vi "Configure Trigger.vi"(8 "error in":errorcluster, 11 "object in":refnum<class "Fetch Waveforms CFG.lvclass">) -> (0 "error out":errorcluster, 3 "object out":refnum<class "Fetch Waveforms CFG.lvclass">)   [LabVIEW 2023, in "Scope Simulated CFGs.lvlib" / "Fetch Waveforms CFG.lvclass"]
uses:
  Fetch Waveforms CFG.lvclass
  Configuration/Configuration JSON/Configuration JSON Base/CFG JSON.lvclass/CFG JSON.ctl
  49d2c016-646b-4808-92bd-86f31724cd2e.vi
  <vilib>/JDP Science/JSONtext/Find Item.vi
  <vilib>/JDP Science/JSONtext/Next JSON Value.vi
  <vilib>/JDP Science/JSONtext/String Subset.vi
  <vilib>/JDP Science/JSONtext/Parsing/Advance past next JSON Value (inlined COPY).vi
  <vilib>/JDP Science/JSONtext/Parsing/Advance past whitespace.vi
  <vilib>/JDP Science/JSONtext/Parsing/Advance past String.vi
  <vilib>/JDP Science/JSONtext/Parsing/Advance past Number.vi
  <vilib>/JDP Science/JSONtext/Parsing/Advance past Line Ending.vi
  <vilib>/JDP Science/JSONtext/Parsing/Parse Full Path or Item Name.vi
  <vilib>/JDP Science/JSONtext/Parsing/Advance past Array.vi
  <vilib>/JDP Science/JSONtext/Parsing/Advance past Object.vi
  <vilib>/JDP Science/JSONtext/support/Error Cluster From Code.vi
  <vilib>/JDP Science/JSONtext/Offset/Find Item Locations by Path.vi
  <vilib>/JDP Science/JSONtext/JSON text to Variant.vi
  <vilib>/Utility/error.llb/Error Cluster From Error Code.vi
  <vilib>/JDP Science/JSONtext/LVClass Serializer/JSONtext LVClass Serializer.lvclass
  <vilib>/ErrorRing/Error Ring.xnode
  Fetch Waveforms CFG.lvclass/Fetch Waveforms CFG.ctl
  Configuration/Configuration JSON/Configuration JSON Base/CFG JSON.lvclass
panel:
  out "Data":T1
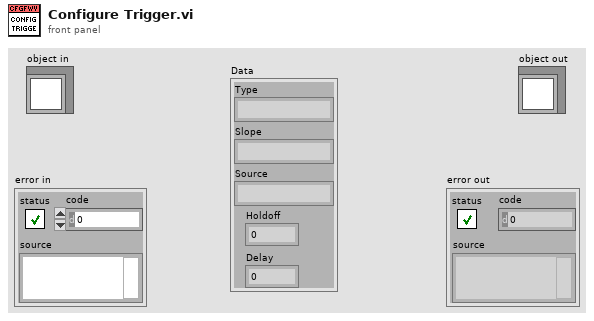
[diagram p1: front panel]
types:
  T1 = cluster{"Type":string, "Slope":string, "Source":string, "Holdoff":dbl, "Delay":dbl}
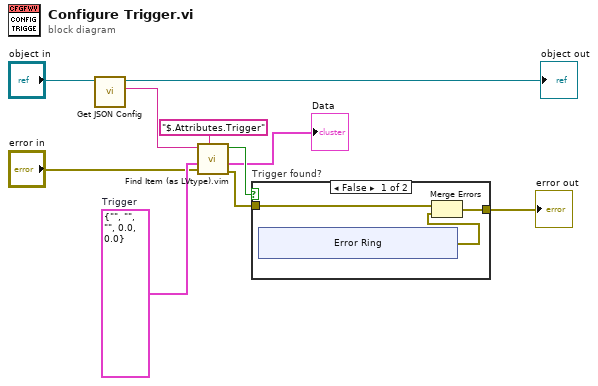
[diagram p0: block diagram]
diagram:
  w8 = T1 {"Type"="", "Slope"="", "Source"="", "Holdoff"=0.0, "Delay"=0.0}  # Trigger
  n1 = call "Get JSON Config.vi"("CFG Base in"="object in") -> ("<JSON>Config>"=w9:string, "CFG Base out"=→"object out":refnum<class "Fetch Waveforms CFG.lvclass">)  [unwired: 9 in]
  n2 = call "Find Item (as LVtype).vim"("$Path or Item Name"="$.Attributes.Trigger", "error in (no error)"="error in", "Data Type and Default Value"=w8, "JSON"=w9) -> ("error out"=w6:errorcluster, "Data"=→"Data":T1, "Found"=w7:bool)  [unwired: 4 in, 1 out]
  n3 = case "Trigger found?" shown="False" w7 {
    tunnel: [w13 w19] -> w3
    tunnel: w6 -> [w11 w19]
    frame False {
      n4 = xnode "Error Ring"() -> ("error out"=w12:errorcluster)
      n5 = Merge Errors(w11, w12) -> (w13:errorcluster)
    }
    frame True {
    }
  }
  "error out" <- w3
